vi "Execute.vi"(7 "Peeping?":bool, 8 "error in (no error)":errorcluster, 9 "Targets":T1[](array[typedef]), 11 "Project Path":path) -> (0 "error out":errorcluster)   [LabVIEW 2025, in "Project.lvclass"]
doc: "Script VI from the CSV configuration."
uses:
  Project.lvclass
  FPGA Settings.ctl
  Module/Module/Module Settings.ctl
  Signal/Signal/Signal Settings.ctl
  Read Folder Ref.vi
  Project.lvclass/Project.ctl
  VI/VI/VI.lvclass
  Signal/Signal/Signal.lvclass
  Module/Module/Module.lvclass
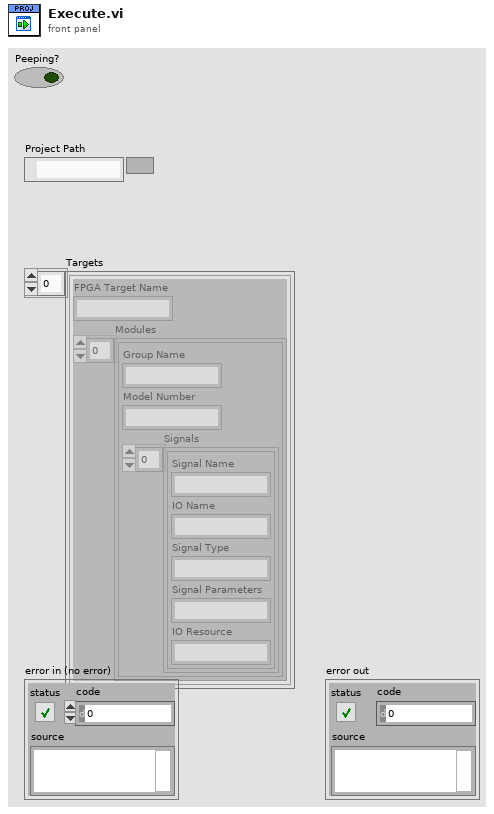
[diagram p1: front panel]
types:
  T1 = typedef "Project.lvclass/FPGA Settings.ctl" = cluster{"FPGA Target Name":string, "Modules":T2[]}
  T2 = typedef "Module.lvclass/Module Settings.ctl" = cluster{"Group Name":string, "Model Number":string, "Signals":T3[]}
  T3 = typedef "Signal.lvclass/Signal Settings.ctl" = cluster{"Signal Name":string, "IO Name":string, "Signal Type":string, "Signal Parameters":string, "IO Resource":string}
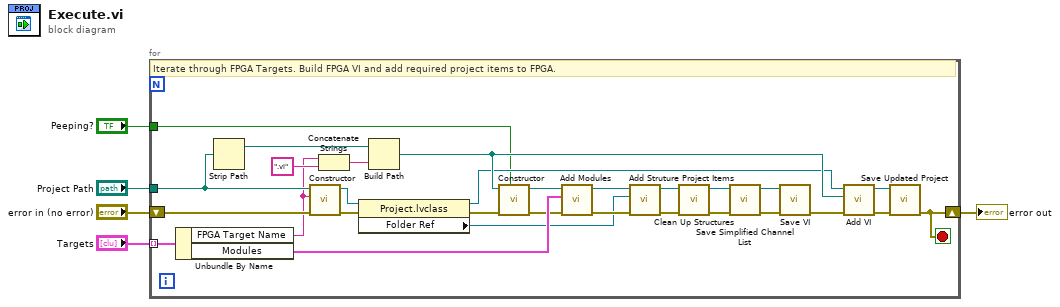
[diagram p0: block diagram]
diagram:
  n1 = for {
    tunnel: "Project Path" -> [w20]
    shift-right: [w7] -> w3
    shift-left: "error in (no error)" -> [w32]
    tunnel: "Targets" -> [w31] mode=indexing
    tunnel: "Peeping?" -> [w6]
    stop <- w7 stop-if-true
    # "Iterate through FPGA Targets. Build FPGA VI and add required project items to FPGA."
    n2 = Unbundle By Name(w31) -> ("FPGA Target Name"=w19:string, "Modules"=w30:T2[])
    n3 = Strip Path(path=w20) -> (stripped path=w22:path)  [unwired: 1 out]
    n4 = call "Constructor.vi"("error in (no error)"=w32, "FPGA Target Name"=w19, "Project Path"=w20) -> ("error out"=w33:errorcluster, "Project out"=w34:refnum<class "Project.lvclass">)  [unwired: 7 in]
    n5 = Concatenate Strings(w19, ".vi" ("string")) -> (w18:string)
    n6 = property class="Project.lvclass"(reference=w34, error in=w33) -> (reference out=w11:refnum<class "Project.lvclass">, error out=w8:errorcluster, "Folder Ref"=w23:refnum<vi>)
    n7 = Build Path(base path=w22, name or relative path=w18) -> (appended path=w13:path)
    n8 = call "Constructor.vi"("Peeping?"=w6, "error in (no error)"=w8, "Path"=w13) -> ("error out"=w27:errorcluster, "Block Diagram"=w26:refnum<class "VI.lvclass">)  [unwired: 7 in]
    n9 = call "Add Modules.vi"("error in (no error)"=w27, "Modules"=w30, "Block Diagram in"=w26) -> ("error out"=w28:errorcluster, "Block Diagram out"=w29:refnum<class "VI.lvclass">)  [unwired: 7 in]
    n10 = call "Add Struture Project Items.vi"("error in (no error)"=w28, "Folder Location Ref"=w23, "Block Diagram in"=w29) -> ("error out"=w25:errorcluster, "Block Diagram out"=w24:refnum<class "VI.lvclass">)  [unwired: 7 in]
    n11 = call "Clean Up Structures.vi"("error in (no error)"=w25, "Block Diagram in"=w24) -> ("error out"=w17:errorcluster, "Block Diagram out"=w16:refnum<class "VI.lvclass">)  [unwired: 8 in]
    n12 = call "Save Simplified Channel List.vi"("error in (no error)"=w17, "VI in"=w16) -> ("error out"=w14:errorcluster, "VI out"=w15:refnum<class "VI.lvclass">)  [unwired: 8 in]
    n13 = call "Save VI.vi"("error in (no error)"=w14, "VI in"=w15) -> ("error out"=w12:errorcluster)  [unwired: 8 in, 1 out]
    n14 = call "Add VI.vi"("error in (no error)"=w12, "Path"=w13, "Project in"=w11) -> ("error out"=w9:errorcluster, "Project out"=w10:refnum<class "Project.lvclass">)  [unwired: 7 in]
    n15 = call-dynamic "Save Updated Project.vi"("error in (no error)"=w9, "Project in"=w10) -> ("error out"=w7:errorcluster)  [unwired: 8 in, 1 out]
  }
  "error out" <- w3
